vi "XML_led.vi"(1 "Testpulse Cluster":T1={"Master Pulser On/Off"=FALSE, "Testpulse Turnaround Time (samples)"=14, "Pulse Separation (samples)"=0, "Pulse duration (samples)"=0}, 2 "Input String":string) -> (0 "Output String":string)   [LabVIEW 2012]
panel:
  in  "Master Pulser On/Off":bool
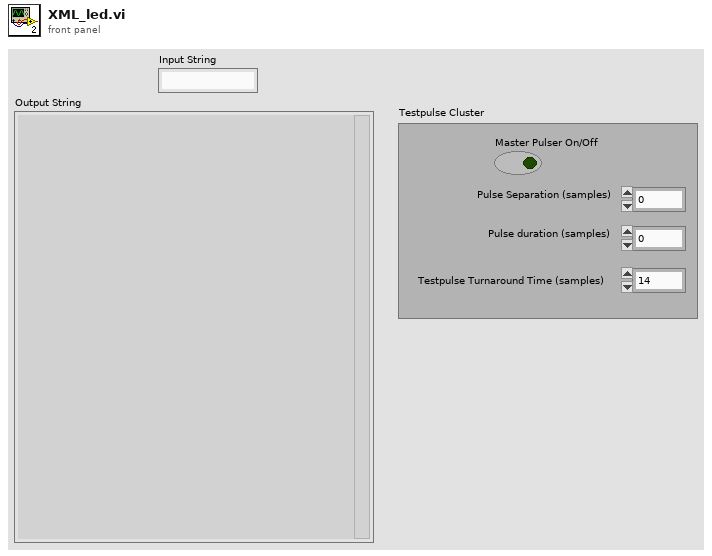
[diagram p1: front panel]
types:
  T1 = cluster{"Master Pulser On/Off":bool, "Testpulse Turnaround Time (samples)":u32, "Pulse Separation (samples)":u32, "Pulse duration (samples)":u32}
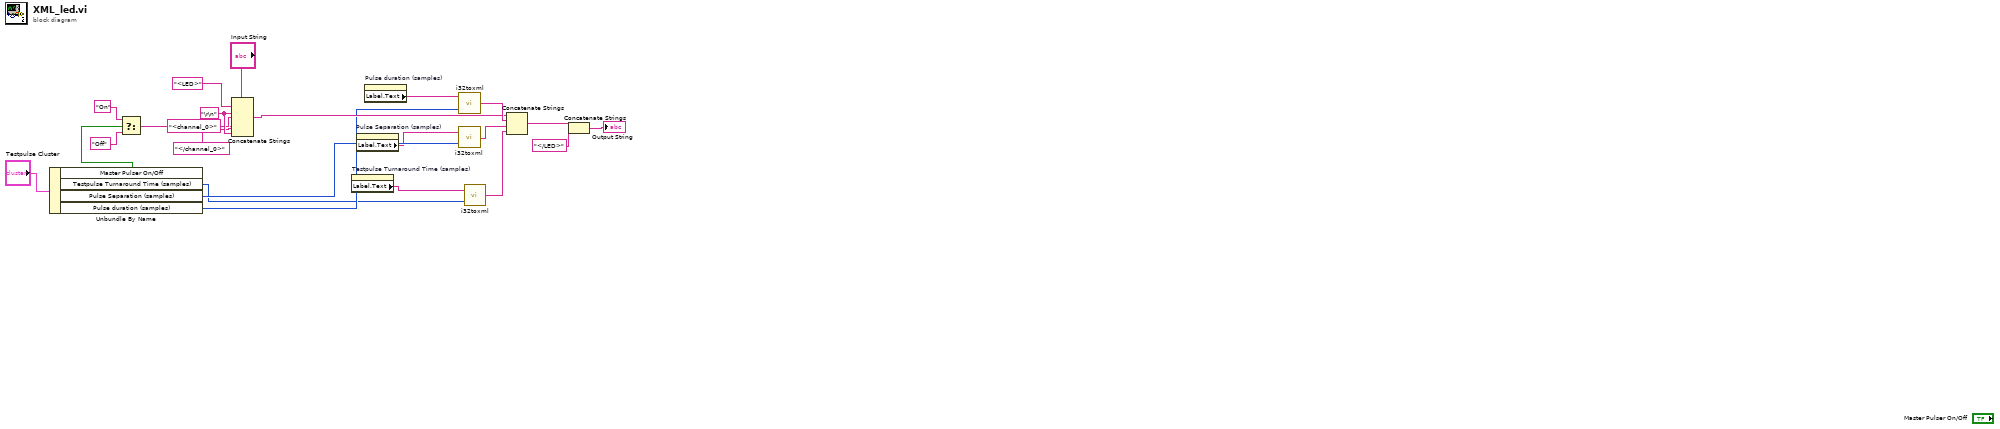
[diagram p0: block diagram]
diagram:
  w17 = "\r\n"
  n1 = Unbundle By Name("Testpulse Cluster") -> ("Master Pulser On/Off"=w7:bool, "Testpulse Turnaround Time (samples)"=w4:u32, "Pulse Separation (samples)"=w5:u32, "Pulse duration (samples)"=w6:u32)
  n2 = Select(t="On", s=w7, f="Off") -> (s? t:f=w9:string)
  n3 = Concatenate Strings("Input String", "<LED>" ("string"), w17, "<channel_0>" ("string"), w9, "</channel_0>" ("string"), w17) -> (w18:string)
  n4 = property on="Testpulse Turnaround Time (samples)" class="DigNum (strict)"() -> ("Label.Text"=w1:string)  [unwired: 2 in, 2 out]
  n5 = property on="Pulse Separation (samples)" class="DigNum (strict)"() -> ("Label.Text"=w2:string)  [unwired: 2 in, 2 out]
  n6 = property on="Pulse duration (samples)" class="DigNum (strict)"() -> ("Label.Text"=w3:string)  [unwired: 2 in, 2 out]
  n7 = call "i32toxml.vi"("variable"=w6, "variable name"=w3) -> ("xml string"=w19:string)
  n8 = call "i32toxml.vi"("variable"=w5, "variable name"=w2) -> ("xml string"=w20:string)
  n9 = call "i32toxml.vi"("variable"=w4, "variable name"=w1) -> ("xml string"=w23:string)
  n10 = Concatenate Strings(w18, w19, w20, w23) -> (w22:string)
  n11 = Concatenate Strings(w22, "</LED>" ("string")) -> (→"Output String":string)
